vi "flow controlled Read Tick.vi"(10 "error in":errorcluster) -> (2 "error out":errorcluster, 3 "millisecond timer value":u32)   [LabVIEW 2023, in "Instruments.lvlib" / "Instruments.lvclass"]
uses:
  Library/Instruments.lvclass
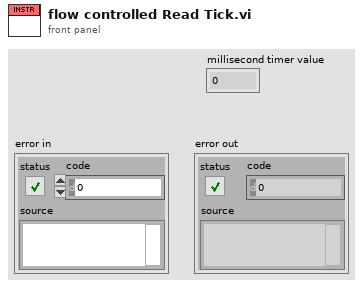
[diagram p1: front panel]
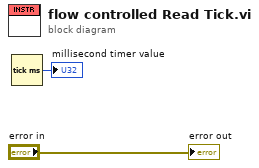
[diagram p0: block diagram]
diagram:
  n1 = Tick Count (ms)() -> (millisecond timer value=→"millisecond timer value":u32)
  "error out" <- "error in"
